vi "MH_DeInit.vi"(8 "error in (no error)":errorcluster, 11 "Multiharp in":refnum<class "Multiharp.lvclass">) -> (0 "error out":errorcluster, 3 "Multiharp out":refnum<class "Multiharp.lvclass">)   [LabVIEW 2023, in "Multiharp.lvlib" / "Multiharp.lvclass"]
uses:
  Multiharp.lvclass
  <vilib>/ActorFramework/Actor/Actor.lvclass
  MultiharpComm Messages/MH_DeInitDone Msg/MH_DeInitDone Msg.lvclass
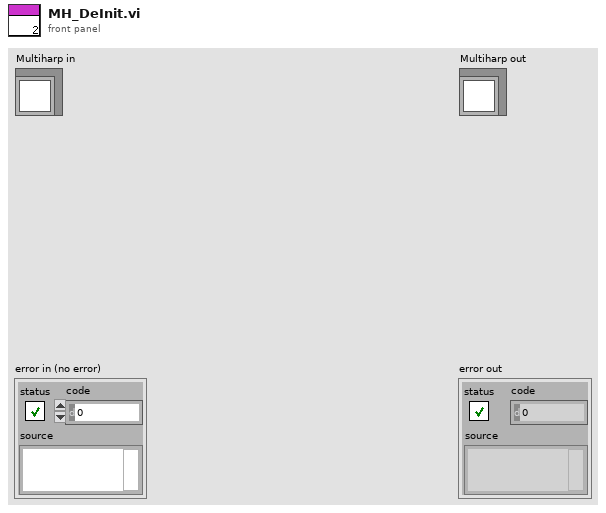
[diagram p1: front panel]
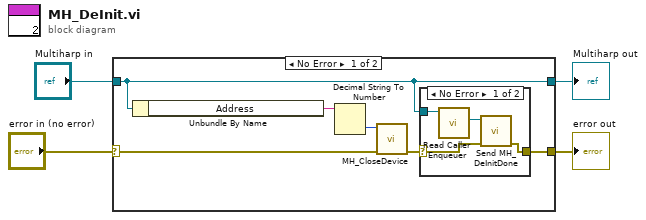
[diagram p0: block diagram]
diagram:
  n1 = case shown="No Error" "error in (no error)" {
    selector: "error in (no error)" -> [w6 w17]
    tunnel: [w5 w17] -> w3
    tunnel: [w10 w16] -> w1
    tunnel: "Multiharp in" -> [w10 w16]
    frame No Error {
      n2 = Unbundle By Name(w10) -> ("Address"=w9:string)
      n3 = Decimal String To Number(string=w9) -> (number=w8:i32)  [unwired: 2 in, 1 out]
      n4 = call "MH_CloseDevice.vi"("error in (no error)"=w6, "devidx"=w8) -> ("error out"=w7:errorcluster)  [unwired: 8 in, 1 out]
      n5 = case shown="No Error" w7 {
        selector: w7 -> [w12 w15]
        tunnel: w10 -> [w14 _]
        tunnel: [w11 w15] -> w5
        frame No Error {
          n6 = call <vilib>:"Read Caller Enqueuer.vi"("Actor"=w14) -> ("Caller Enqueuer"=w13:refnum<class "Message Enqueuer.lvclass">)  [unwired: 10 in]
          n7 = call "Send MH_DeInitDone.vi"("error in (no error)"=w12, "Message Enqueuer"=w13) -> ("error out"=w11:errorcluster)  [unwired: 8 in, 1 out]
        }
        frame Error {
        }
      }
    }
    frame Error {
    }
  }
  "error out" <- w3
  "Multiharp out" <- w1
